vi "Remove Topic.vi"(8 "error in (no error)":errorcluster, 10 "Topic":refnum<class "Topic.lvclass">, 11 "TopicLookupTable":refnum<data-value>) -> (0 "error out":errorcluster, 3 "TopicLookupTable":refnum<data-value>)   [LabVIEW 2015, in "Mediator.lvlib" / "TopicLookupTable.lvclass"]
doc: "<License>\nCopyright © 2017 Composed Systems, LLC | All rights reserved\nwww.composed.io\n\nAuthor: Ethan Stern <ethan.stern@composed.io>\n\nThis software is provided \"AS IS\" WITHOUT WARRANTIES, either express or implied, AND IS FOR EDUCATIONAL PURPOSES ONLY.\n</License>"
uses:
  TopicLookupTable.lvclass
  Topic/Topic.lvclass
  TopicLookupTable.lvclass/TopicLookupTable.ctl
  Topic/Topic.lvclass/Topic.ctl
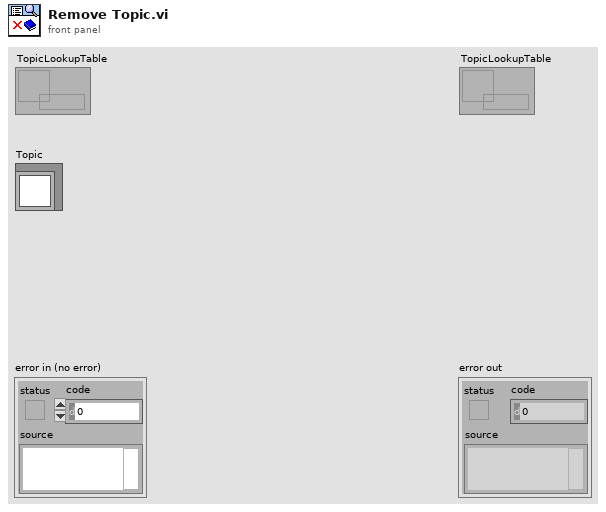
[diagram p1: front panel]
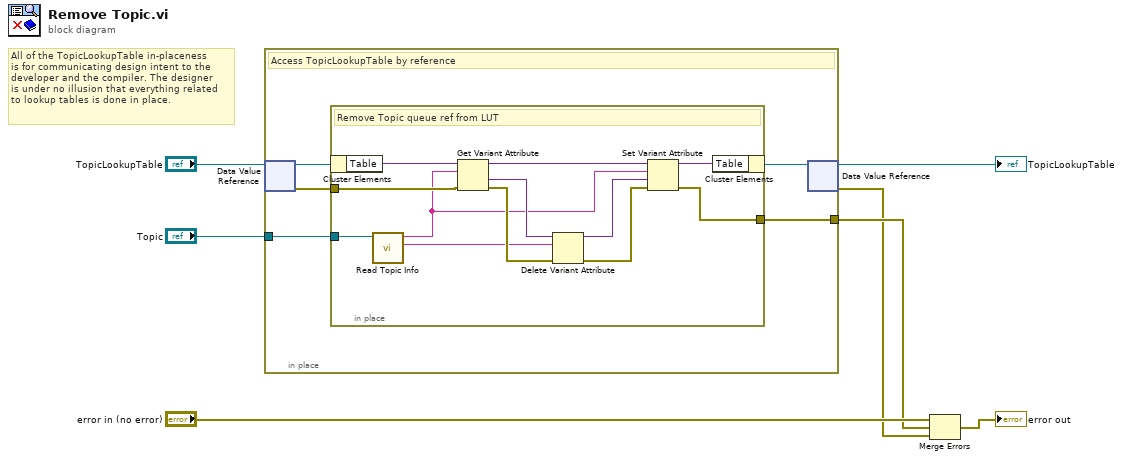
[diagram p0: block diagram]
diagram:
  # "All of the TopicLookupTable in-placeness\nis for communicating design intent to the\ndeveloper and the compiler. The designer\nis under no illusion that everything related\nto lookup tables is done in place."
  n1 = in-place {
    in-place-border: [w12] -> w5
    in-place-border: "Topic" -> [w11]
    # "Access TopicLookupTable by reference"
    n2 = in-place-dvr #1("TopicLookupTable") -> (w10:refnum<class "TopicLookupTable.lvclass">, w8:errorcluster)
    n3 = in-place {
      in-place-border: [w21] -> w12
      in-place-border: w11 -> [w20]
      in-place-border: w8 -> [w23]
      # "Remove Topic queue ref from LUT"
      n4 = in-place-cluster #2(w10) -> ("Table"=w19:variant)
      n5 = call "Read Topic Info.vi"("Topic in"=w20) -> ("Name"=w14:string, "Type"=w13:string)  [unwired: 7 in, 2 out]
      n6 = Get Variant Attribute(Variant=w19, name=w13, error in=w23) -> (duplicate Variant=w18:variant, value=w17:variant, error out=w24:errorcluster)  [unwired: 1 in, 1 out]
      n7 = Delete Variant Attribute(4:w24, 6:w14, 7:w17) -> (0:w15:errorcluster, 3:w16:variant)  [unwired: 1 out]
      n8 = Set Variant Attribute(Variant=w18, name=w13, value=w16, error in=w15) -> (Variant out=w22:variant, error out=w21:errorcluster)  [unwired: 1 out]
      n9 = in-place-cluster #2("Table"=w22) -> (w9:refnum<class "TopicLookupTable.lvclass">)
    }
    n10 = in-place-dvr #1(w9) -> (→"TopicLookupTable":refnum<data-value>, w2:errorcluster)
  }
  n11 = Merge Errors("error in (no error)", w5, w2) -> (→"error out":errorcluster)
